vi "HIDRA.vi"() -> ()   [LabVIEW 2017]
uses:
  Type_Defs/Control.ctl
  Type_Defs/Diagnostics.ctl
  Type_Defs/Systems.ctl
  Type_Defs/Data.ctl
  Type_Defs/States.ctl
panel:
  out "Data Collecting?":bool
  in  "Data":T1
  out "Pressure":dbl format="%#.3g"
  out "Systems":T3
  out "Experiment State":T4(ring)
  out "Experiment Purpose":string
  out "Diagnostics":T2
  out "Step Number":i32
  out "Current Step Instructions":string
  in  "Controls":T5
  out "Time Elapsed":string
  out "Current Time":timestamp format="%<%X\n%x>T"
  out "Start Time":timestamp format="%<%X\n%x>T"
  out "Experiment Number":i32
  out "Operator":string
  # "HIDRA Control System"
  # "User Controls"
  # "Diagnostics"
  # "IGNORE PRESSURE AND SYSTEMS READINGS; NOT SET UP YET"
  # "Experiment Information"
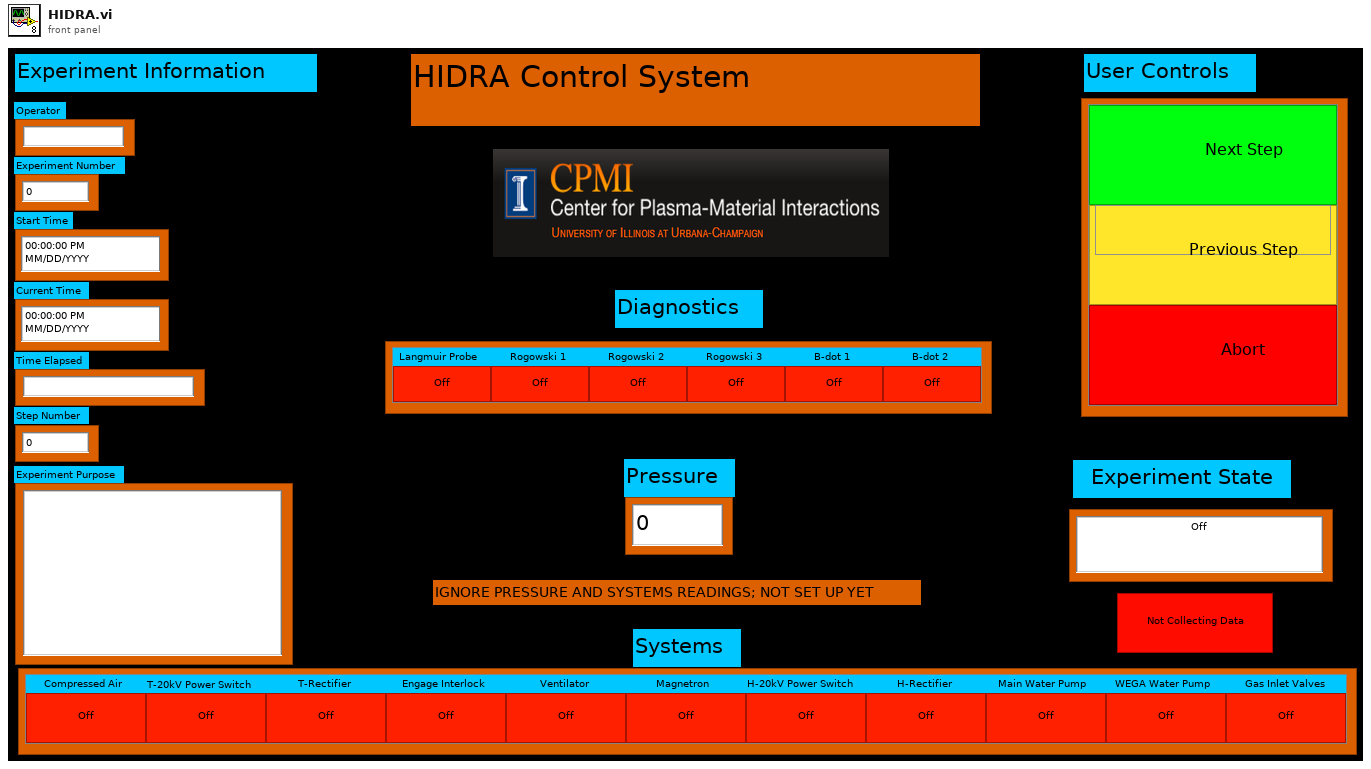
[diagram p1: front panel]
types:
  T1 = typedef "Data.ctl" = cluster{"User Name":string, "Experiment Number":i32, "Start Time":timestamp, "Data":dbl[], "Step Number":i32, "Step Instructions":string, "Diagnostics":T2, "Experiment Purpose":string, "Experiment State":enum16{"Off", "Setting Up", "Ready", "In Progress", "Shutting Down"}, "Systems":T3, "Vacuum Pressure":dbl, "Fieldpoints":cluster{"System Boolean Fieldpoints":cluster{"Compressed Air":refnum<k21>, "T-20kV Power Switch":refnum<k21>, "T-Rectifier":refnum<k21>, "Engage Interlock":refnum<k21>, "Ventilator":refnum<k21>, "Magnetron":refnum<k21>, "H-20kV Power Switch":refnum<k21>, "H-Rectifier":refnum<k21>, "Main Water Pump":refnum<k21>, "WEGA Water Pump":refnum<k21>, "Gas Inlet Valves":refnum<k21>}, "Step Fieldpoints":cluster{"Exhaust Ventillator":refnum<k21>, "Compressed Air":refnum<k21>, "Water Pressure":refnum<k21>, "Interlock":refnum<k21>, "Toroidal Power Supply 1":refnum<k21>, "Toroidal Power Supply 2":refnum<k21>, "Toroidal Rectifier":refnum<k21>, "Helical Power Supply":refnum<k21>, "Helical Rectifier":refnum<k21>, "6kW Magnetron Standby":refnum<k21>, "20kW Magnetron Standby":refnum<k21>}}, "Pressure History":cluster{"Seconds into Experiment":i32[], "Pressure Data":dbl[]}, "Time Computer Control":dbl[], "Toroidal Voltage Computer Control":dbl[], "Helical Voltage Computer Control":dbl[], "Toroidal Current":dbl[], "Toroidal Voltage":dbl[], "Toroidal Current Set Point":dbl[], "Helical Current Set Point":dbl[], "Helical Voltage":dbl[], "Helical Current":dbl[], "Experiment Folder":path, "Run Another Shot?":bool}
  T2 = typedef "Diagnostics.ctl" = cluster{"Langmuir Probe":bool, "Rogowski 1":bool, "Rogowski 2":bool, "Rogowski 3":bool, "B-dot 1":bool, "B-dot 2":bool}
  T3 = typedef "Systems.ctl" = cluster{"Compressed Air":bool, "T-20kV Power Switch":bool, "T-Rectifier":bool, "Engage Interlock":bool, "Ventilator":bool, "Magnetron":bool, "H-20kV Power Switch":bool, "H-Rectifier":bool, "Main Water Pump":bool, "WEGA Water Pump":bool, "Gas Inlet Valves":bool}
  T4 = enum16{"Off", "Setting Up", "Ready", "In Progress", "Shutting Down"}
  T5 = typedef "Control.ctl" = cluster{"Next Step":bool, "Previous Step":bool, "Abort":bool}
  T6 = typedef "States.ctl" = enum16{"1. Initialize", "2. User Information", "3. Experiment Information", "4. Create Data File", "5. Steps for Setup", "6. Gather Data", "7. Write to Data File", "8. Final", "Stop Pressed - Shutdown State"}
  T7 = enum8{"Enabled", "Disabled", "Disabled and Grayed Out"}
  T8 = enum32{"Invalid", "Standard", "Closed", "Hidden", "Minimized", "Maximized"}
  T9 = enum16{"open", "replace", "create", "open or create", "replace or create", "replace or create with confirmation"}
  T10 = enum16{"Always On", "Always Off", "Off While Running"}
  T11 = cluster{"Seconds into Experiment":i32[], "Pressure Data":dbl[]}
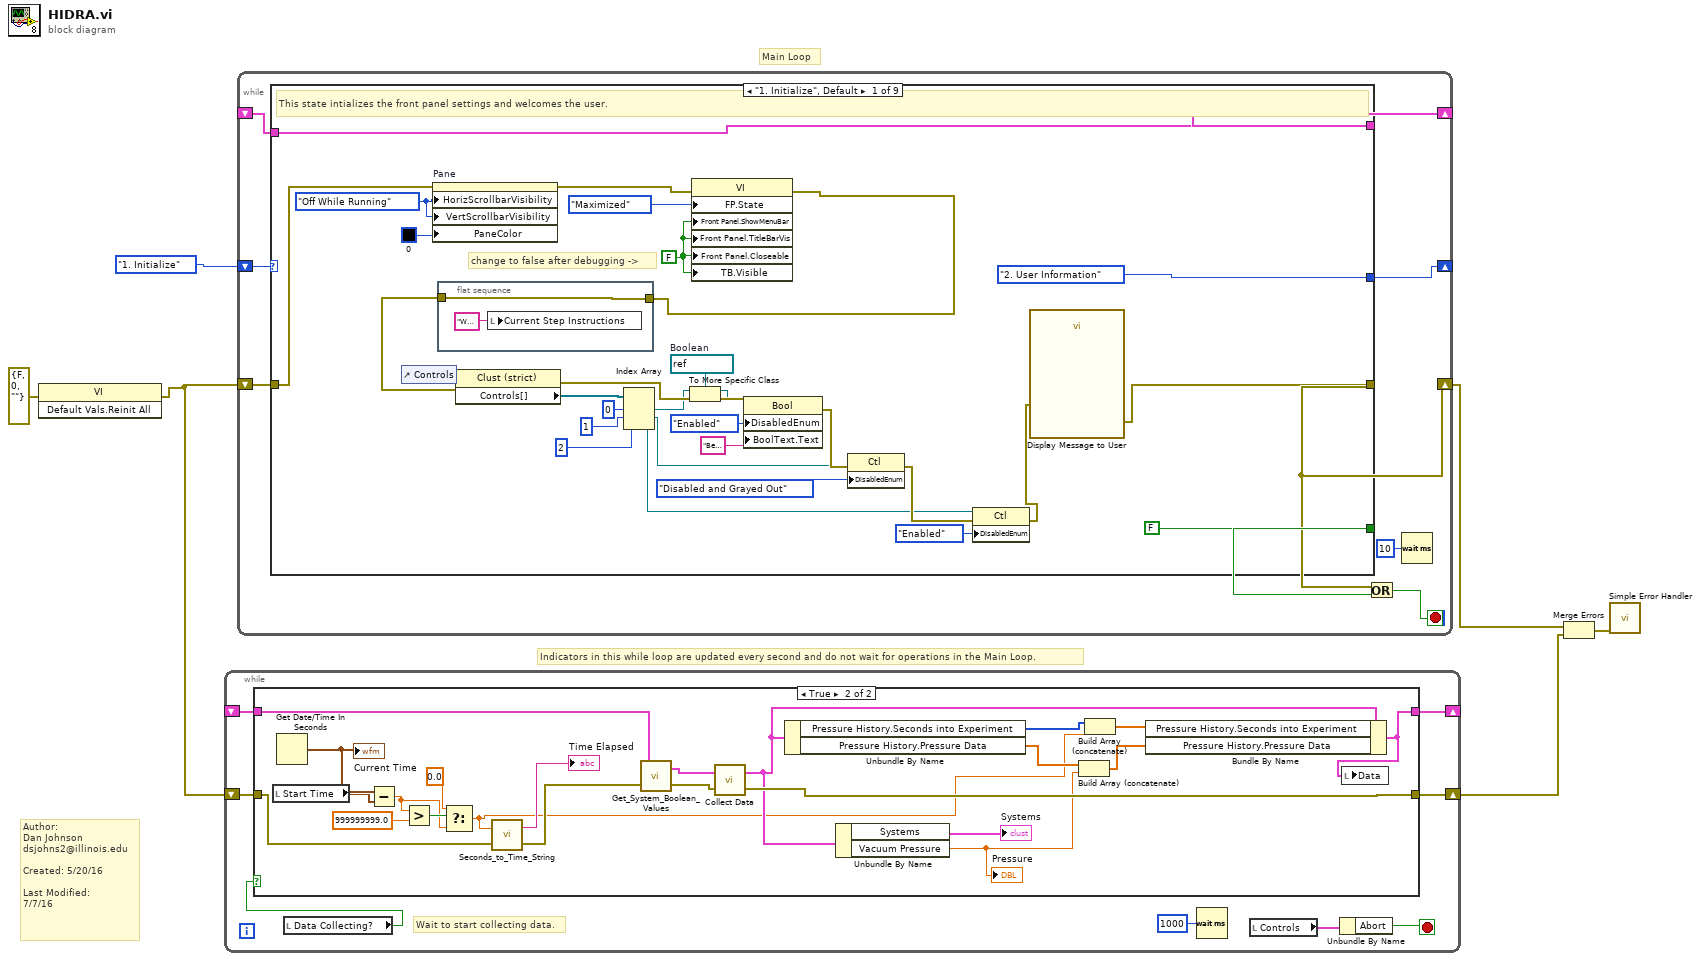
[diagram p0: block diagram]
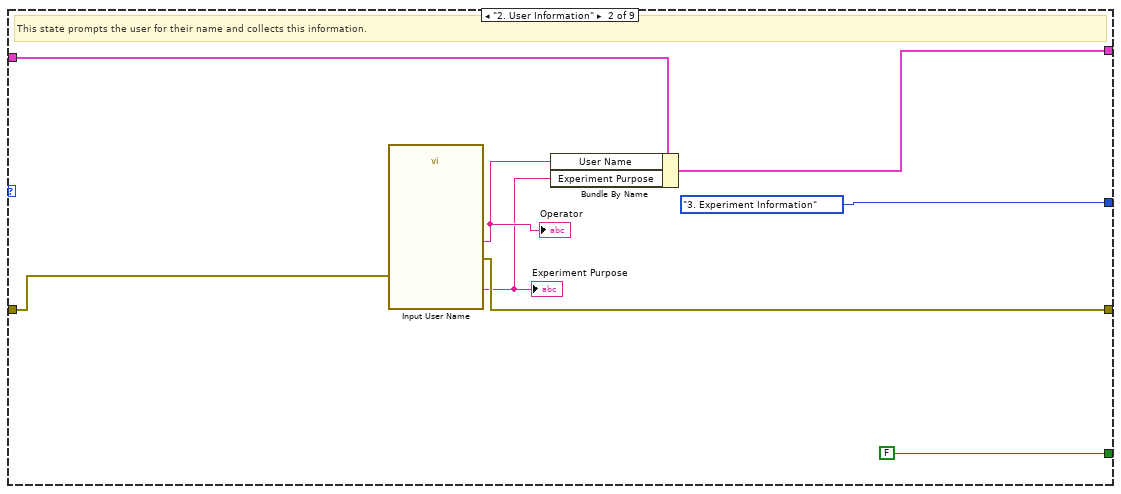
[diagram p3: hidden frame]
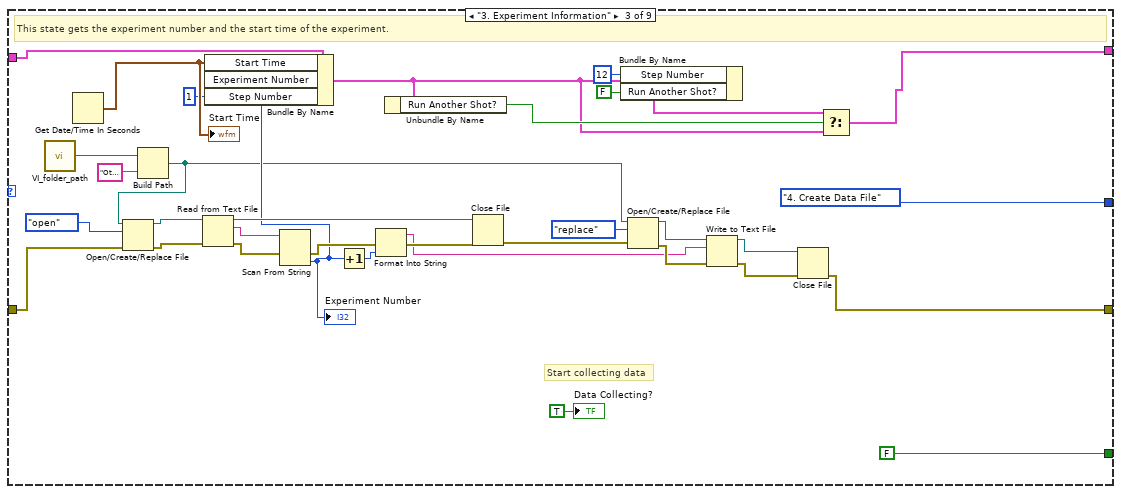
[diagram p4: hidden frame]
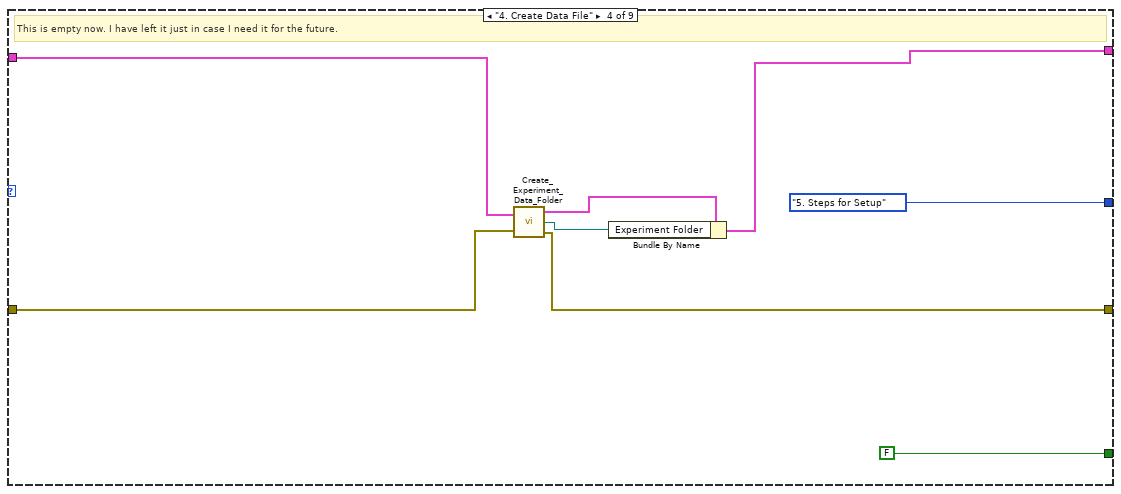
[diagram p5: hidden frame]
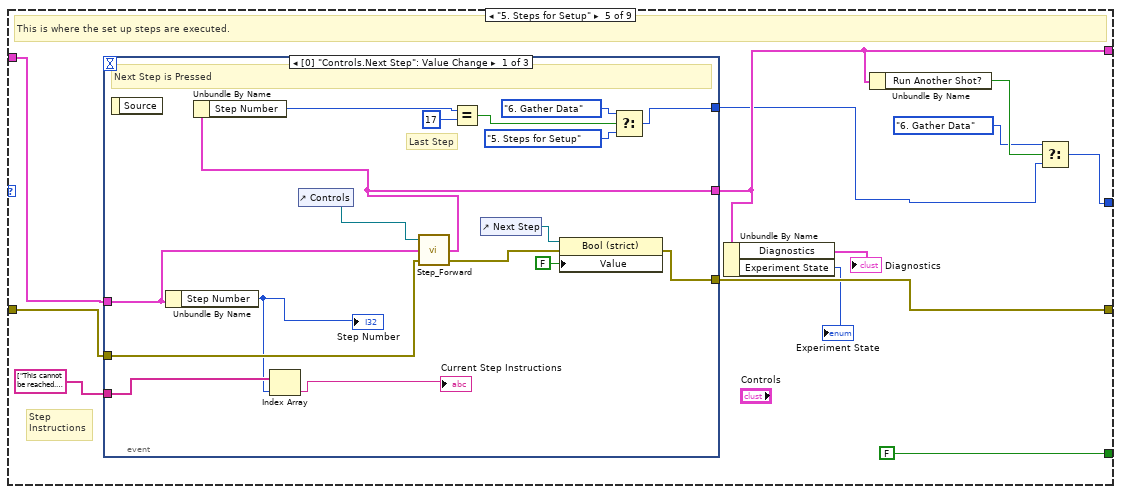
[diagram p6: hidden frame]
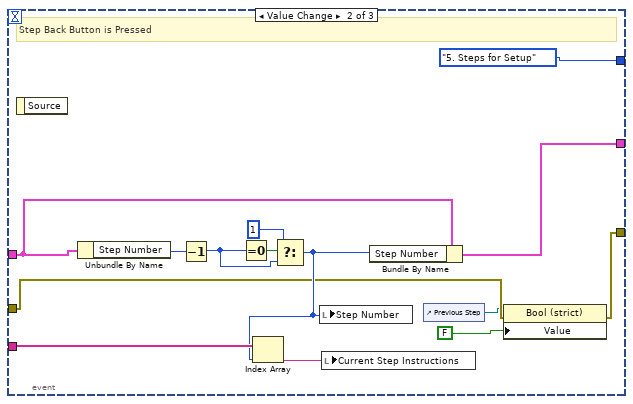
[diagram p7: hidden frame]
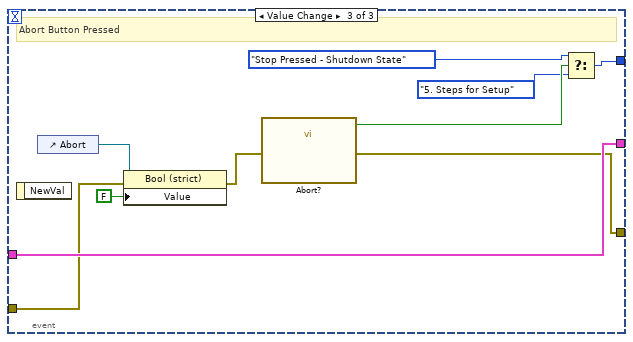
[diagram p8: hidden frame]
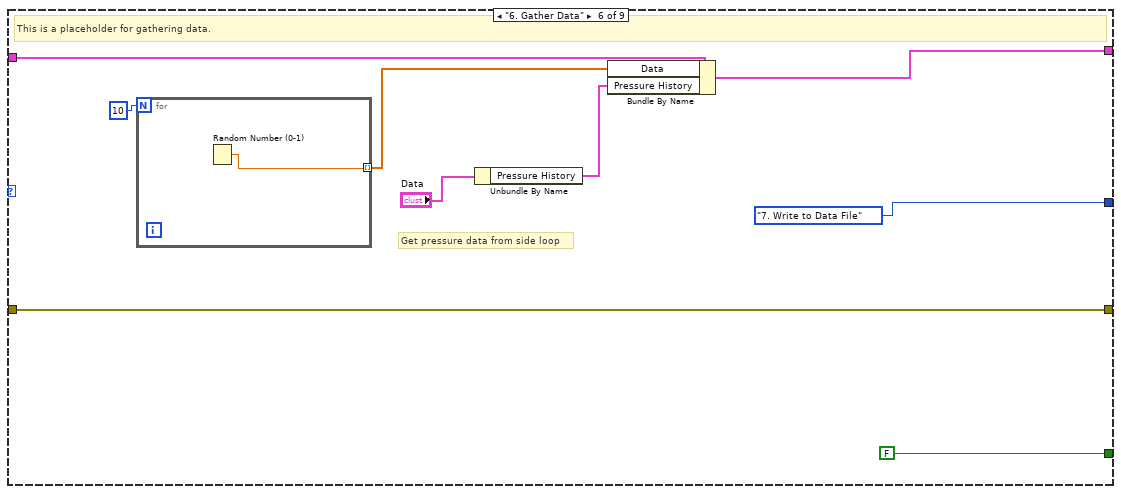
[diagram p9: hidden frame]
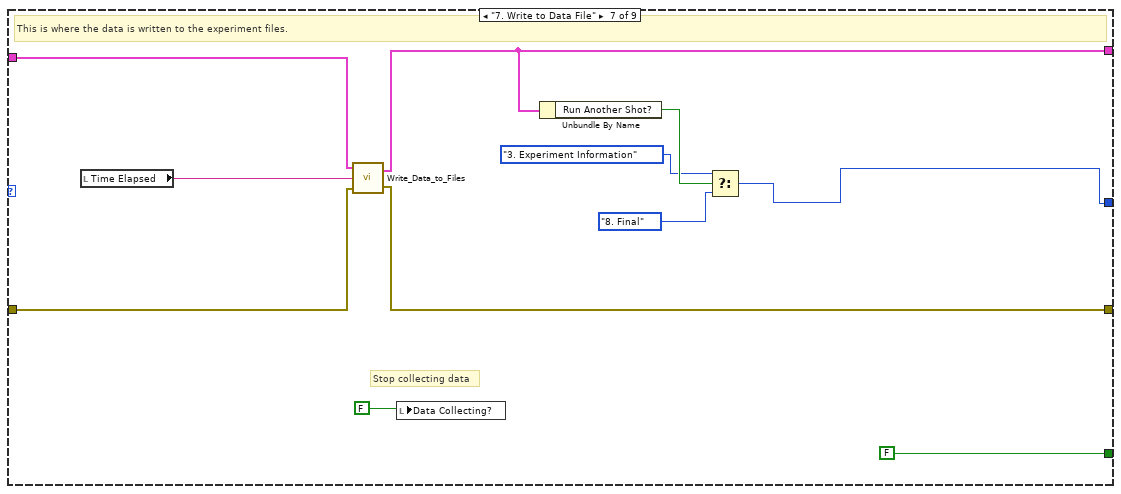
[diagram p10: hidden frame]
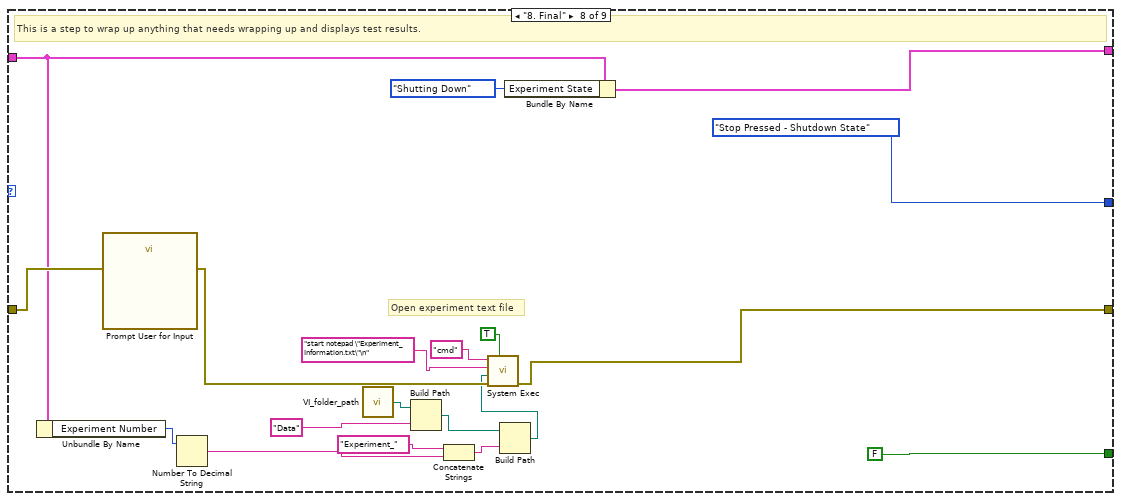
[diagram p11: hidden frame]
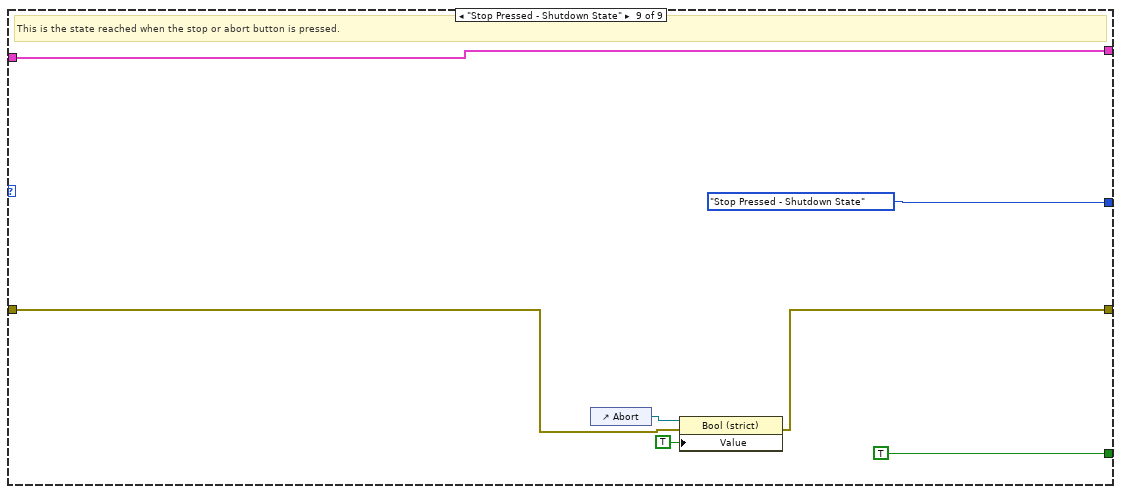
[diagram p12: hidden frame]
diagram:
  # "Main Loop"
  # "Indicators in this while loop are updated every second and do not wait for operations in the Main Loop."
  # "Author:\nDan Johnson\ndsjohns2@illinois.edu\n\nCreated: 5/20/16\n\nLast Modified:\n7/7/16"
  n1 = invoke class="VI" method="Default Vals.Reinit All"(error in=errorcluster {"status"=FALSE, "code"=0, "source"=""} ("error in (no error)")) -> (error out=w2:errorcluster)  [unwired: 2 in, 2 out]
  n2 = while {
    shift-right: [w13] -> w4
    shift-left: w2 -> [w12]
    shift-right: [w8] -> _
    shift-left: _ -> [w9]
    stop <- w10 stop-if-true
    # "Wait to start collecting data."
    n3 = local read "Data Collecting?"() -> (w7:bool)
    n4 = case shown="True" w7 {
      tunnel: [w16 w35] -> w13
      tunnel: w12 -> [w16 w18]
      tunnel: w9 -> [w15 w26]
      tunnel: [w15 w24] -> w8
      frame False {
      }
      frame True {
        n5 = local read "Start Time"() -> (w32:timestamp)
        n6 = Get Date/Time In Seconds() -> (seconds since 1Jan1904=w33:timestamp)
        "Current Time" <- w33
        n7 = Subtract(x=w33, y=w32) -> (x-y=w28:dbl)
        n8 = Greater?(x=w28, y=999999999.0) -> (0:w29:bool)
        n9 = Select(t=0.0, s=w29, f=w28) -> (s? t:f=w17:dbl)
        n10 = call "Seconds_to_Time_String.vi"("error in"=w18, "Seconds in"=w17) -> ("error out"=w34:errorcluster, "String"=→"Time Elapsed":string)
        n11 = call "Get_System_Boolean_Values.vi"("error in"=w34, "Data in"=w26) -> ("error out"=w37:errorcluster, "Data out"=w38:T1)
        n12 = call "Collect Data.vi"("error constant"=w37, "Data in"=w38) -> ("error constant 2"=w35:errorcluster, "Data out"=w25:T1)
        n13 = Unbundle By Name(w25) -> ("Pressure History.Seconds into Experiment"=w23:i32[], "Pressure History.Pressure Data"=w20:dbl[])
        n14 = Unbundle By Name(w25) -> ("Systems"=→"Systems":T3, "Vacuum Pressure"=w19:dbl)
        "Pressure" <- w19
        n15 = Build Array (concatenate)(w20, w19) -> (w21:dbl[])
        n16 = Build Array (concatenate)(w23, w17) -> (w22:dbl[])
        n17 = Bundle By Name(cluster=w25, "Pressure History.Seconds into Experiment"=w22, "Pressure History.Pressure Data"=w21) -> (w24:T1)
        n18 = local write "Data"(w24) -> ()
      }
    }
    n19 = Wait (ms)(milliseconds to wait=u32 1000) -> ()  [unwired: 1 out]
    n20 = local read "Controls"() -> (w11:T5)
    n21 = Unbundle By Name(w11) -> ("Abort"=w10:bool)
  }
  n22 = while {
    shift-right: [w39] -> _
    shift-left: States."1. Initialize" ("Enum") -> [w41]
    shift-right: [w40] -> _
    shift-left: _ -> [w46]
    shift-right: [w42] -> w5
    shift-left: w2 -> [w47]
    stop <- w44 stop-if-true
    n23 = case shown="\"1. Initialize\", Default" w41 {
      tunnel: w47 -> [w72 w86 w120 w127 w137 w186 w202 w219 w224]
      tunnel: w46 -> [w78 w84 w101 w128 w141 w191 w200 w214 w229]
      tunnel: [w78 w83 w93 w124 w135 w187 w196 w221 w229] -> w40
      tunnel: [FALSE FALSE FALSE FALSE FALSE FALSE FALSE FALSE TRUE] -> w43
      tunnel: [w71 w85 w100 w126 w140 w186 w201 w205 w225] -> w42
      tunnel: [States."2. User Information" ("Enum") States."3. Experiment Information" ("Enum") States."4. Create Data File" ("Enum") States."5. Steps for Setup" ("Enum") w131 States."7. Write to Data File" ("Enum") w194 States."Stop Pressed - Shutdown State" ("Enum") States."Stop Pressed - Shutdown State" ("Enum")] -> w39
      frame "1. Initialize", Default {
        w50 = refnum<vi> refnum  # Boolean
        w70 = FALSE
        w74 = T10."Off While Running" ("Vertical Scrollbar Visibility")
        # "change to false after debugging ->"
        # "This state intializes the front panel settings and welcomes the user."
        n24 = control-ref of="Controls"() -> (w68:refnum<vi>)
        n25 = property on="Pane" class="Pane"(error in=w72, "HorizScrollbarVisibility"=w74, "VertScrollbarVisibility"=w74, "PaneColor"=u32 0) -> (error out=w75:errorcluster)  [unwired: 1 in, 1 out]
        n26 = flat-sequence {
          tunnel: [w80] -> w55
          tunnel: w48 -> [w80]
          frame #0 {
            n27 = local write "Current Step Instructions"("Welcome to the Hybrid Illinois Device for Research and Applications (HIDRA)!" ("Current Step Instructions")) -> ()
          }
        }
        n28 = property class="Clust (strict)"(reference=w68, error in=w55) -> (error out=w54:errorcluster, "Controls[]"=w57:refnum<vi>[])  [unwired: 1 out]
        n29 = Index Array(array=w57, index #1=0 ("index"), index #2=1 ("index"), index #3=2 ("index")) -> (element #1=w52:refnum<vi>, element #2=w61:refnum<vi>, element #3=w62:refnum<vi>)
        n30 = To More Specific Class(target class=w50, reference=w52, error in=w54) -> (specific class reference=w51:refnum<vi>, error out=w53:errorcluster)
        n31 = property class="VI"(error in=w75, "FP.State"=T8."Maximized" ("Front Panel Window:State"), "Front Panel.ShowMenuBar"=w70, "Front Panel.TitleBarVis"=w70, "Front Panel.Closeable"=w70, "TB.Visible"=w70) -> (error out=w48:errorcluster)  [unwired: 1 in, 1 out]
        n32 = property class="Bool"(reference=w51, error in=w53, "DisabledEnum"=T7."Enabled" ("Disabled"), "BoolText.Text"="Begin Setup Steps" ("Boolean Text.Text")) -> (error out=w63:errorcluster)  [unwired: 1 out]
        n33 = property class="Ctl"(reference=w61, error in=w63, "DisabledEnum"=T7."Disabled and Grayed Out" ("Disabled")) -> (error out=w64:errorcluster)  [unwired: 1 out]
        n34 = property class="Ctl"(reference=w62, error in=w64, "DisabledEnum"=T7."Enabled" ("Disabled")) -> (error out=w56:errorcluster)  [unwired: 1 out]
        n35 = call "Display Message to User"("error in (no error)"=w56) -> ("error out"=w71:errorcluster)  [unwired: 9 in, 1 out]
      }
      frame "2. User Information" {
        # "This state prompts the user for their name and collects this information."
        n36 = call "Input User Name"("error in (no error)"=w86) -> ("Experiment Purpose"=w81:string, "User Name"=w88:string, "error out"=w85:errorcluster)  [unwired: 15 in, 1 out]
        "Operator" <- w88
        "Experiment Purpose" <- w81
        n37 = Bundle By Name(cluster=w84, "User Name"=w88, "Experiment Purpose"=w81) -> (w83:T1)
      }
      frame "3. Experiment Information" {
        # "Start collecting data"
        # "This state gets the experiment number and the start time of the experiment."
        n38 = call "VI_folder_path.vi"() -> ("output path"=w99:path)
        n39 = Get Date/Time In Seconds() -> (seconds since 1Jan1904=w103:timestamp)
        "Start Time" <- w103
        n40 = Build Path(base path=w99, name or relative path="Other\\Experiment_Number.txt") -> (appended path=w97:path)
        n41 = Open/Create/Replace File(file path (use dialog)=w97, error in=w120, operation (0:open)=T9."open") -> (refnum out=w112:refnum<file>, error out=w119:errorcluster)  [unwired: 3 in, 1 out]
        n42 = Read from Text File(file (use dialog)=w112, error in=w119) -> (refnum out=w111:refnum<file>, text=w107:string, error out=w118:errorcluster)  [unwired: 2 in, 1 out]
        n43 = Scan From String(input string=w107, error in=w118) -> (error out=w117:errorcluster, output 1=w104:i32)  [unwired: 3 in, 2 out]
        "Experiment Number" <- w104
        n44 = Bundle By Name(cluster=w101, "Start Time"=w103, "Experiment Number"=w104, "Step Number"=1) -> (w91:T1)
        n45 = Increment(x=w104) -> (x+1=w106:i32)
        n46 = Format Into String(error in=w117, w106) -> (resulting string=w105:string, error out=w116:errorcluster)  [unwired: 2 in]
        n47 = Unbundle By Name(w91) -> ("Run Another Shot?"=w94:bool)
        n48 = Close File(refnum=w111, error in=w116) -> (error out=w115:errorcluster)  [unwired: 1 out]
        n49 = Bundle By Name(cluster=w91, "Step Number"=12, "Run Another Shot?"=FALSE) -> (w92:T1)
        n50 = Open/Create/Replace File(file path (use dialog)=w97, error in=w115, operation (0:open)=T9."replace") -> (refnum out=w110:refnum<file>, error out=w114:errorcluster)  [unwired: 3 in, 1 out]
        n51 = Write to Text File(file (use dialog)=w110, text=w105, error in=w114) -> (refnum out=w109:refnum<file>, error out=w113:errorcluster)  [unwired: 1 in, 1 out]
        n52 = Close File(refnum=w109, error in=w113) -> (error out=w100:errorcluster)  [unwired: 1 out]
        n53 = Select(t=w92, s=w94, f=w91) -> (s? t:f=w93:T1)
        "Data Collecting?" <- TRUE ("Is Data")
      }
      frame "4. Create Data File" {
        # "This is empty now. I have left it just in case I need it for the future."
        n54 = call "Create_Experiment_Data_Folder.vi"("Data in"=w128, "error in"=w127) -> ("Data out"=w125:T1, "Folder path"=w123:path, "error out"=w126:errorcluster)
        n55 = Bundle By Name(cluster=w125, "Experiment Folder"=w123) -> (w124:T1)
      }
      frame "5. Steps for Setup" {
        # "Step\nInstructions"
        # "This is where the set up steps are executed."
        n56 = event shown="[0] \"Controls.Next Step\": Value Change" {
          selector: _ -> [_ _ _]
          dyn-events: _ -> [_ _ _]
          timeout: _ -> [_ _ _]
          tunnel: [w143 States."5. Steps for Setup" ("Enum") w181] -> w132
          tunnel: [w151 w163 w182] -> w140
          tunnel: w141 -> [w157 w172 w183]
          tunnel: [w155 w171 w183] -> w135
          tunnel: string[] ["This cannot be reached.", "This step sets up the step controls.", "Select the Diagnostics to be used.", "This step checks that the Vacuum Pressure is at the right value.", "This step checks that exhaust ventillator is operational.", "This step checks that the compressed air pressure is high enough.", "This step checks that the water pressure is high enough.", "This step checks that the interlock is on.", "This step checks that the toroidal power supply is on.", "This step checks that the toroidal rectifier is on.", "This step checks that the helical power supply is on.", "This step checks that the helical rectifier is on.", "This step sets the magnetron to standby mode.", "This step performs a final check to make sure everything is ready.", "This step does the following:\n  -Starts the Ramp Generator\n  -Opens the Gas Valve\n  -Resets the Radiation Detector", "This step sets up the pulse.", "This step is the pulse."] ("array") -> [w159 w169 _]
          tunnel: w137 -> [w156 w162 w177]
          event Value Change {
            # "Last Step"
            # "Next Step is Pressed"
            n57 = event-data() -> ()  [unwired: 1 in, 1 out]
            n58 = Unbundle By Name(w157) -> ("Step Number"=w154:i32)
            "Step Number" <- w154
            n59 = Index Array(array=w159, index=w154) -> (element=→"Current Step Instructions":string)
            n60 = control-ref of="Controls"() -> (w158:refnum<vi>)
            n61 = call "Step_Forward.vi"("error in"=w156, "Data in"=w157, "Step control reference in"=w158) -> ("error out"=w152:errorcluster, "Data out"=w155:T1)  [unwired: 1 out]
            n62 = Unbundle By Name(w155) -> ("Step Number"=w147:i32)
            n63 = Equal?(x=w147, y=17) -> (x = y?=w146:bool)
            n64 = control-ref of="Next Step"() -> (w150:refnum<vi>)
            n65 = property class="Bool (strict)"(reference=w150, error in=w152, "Value"=FALSE) -> (error out=w151:errorcluster)  [unwired: 1 out]
            n66 = Select(t=States."6. Gather Data" ("Enum"), s=w146, f=States."5. Steps for Setup" ("Enum")) -> (s? t:f=w143:T6)
          }
          event Value Change {
            # "Step Back Button is Pressed"
            n67 = event-data() -> ()  [unwired: 1 in, 1 out]
            n68 = Unbundle By Name(w172) -> ("Step Number"=w173:i32)
            n69 = Decrement(x=w173) -> (x-1=w165:i32)
            n70 = Equal To 0?(x=w165) -> (x = 0?=w167:bool)
            n71 = Select(t=1, s=w167, f=w165) -> (s? t:f=w164:i32)
            n72 = Index Array(array=w169, index=w164) -> (element=w170:string)
            n73 = local write "Step Number"(w164) -> ()
            n74 = local write "Current Step Instructions"(w170) -> ()
            n75 = Bundle By Name(cluster=w172, "Step Number"=w164) -> (w171:T1)
            n76 = control-ref of="Previous Step"() -> (w160:refnum<vi>)
            n77 = property class="Bool (strict)"(reference=w160, error in=w162, "Value"=FALSE) -> (error out=w163:errorcluster)  [unwired: 1 out]
          }
          event Value Change {
            # "Abort Button Pressed"
            n78 = event-data() -> ()  [unwired: 1 in, 1 out]
            n79 = control-ref of="Abort"() -> (w175:refnum<vi>)
            n80 = property class="Bool (strict)"(reference=w175, error in=w177, "Value"=FALSE) -> (error out=w176:errorcluster)  [unwired: 1 out]
            n81 = call "Abort?"("error in (no error)"=w176) -> ("Abort"=w180:bool, "error out"=w182:errorcluster)  [unwired: 17 in]
            n82 = Select(t=States."Stop Pressed - Shutdown State" ("Enum"), s=w180, f=States."5. Steps for Setup") -> (s? t:f=w181:T6)
          }
        }
        n83 = Unbundle By Name(w135) -> ("Diagnostics"=→"Diagnostics":T2, "Experiment State"=→"Experiment State":T4)
        n84 = Unbundle By Name(w135) -> ("Run Another Shot?"=w134:bool)
        n85 = Select(t=States."6. Gather Data" ("Enum"), s=w134, f=w132) -> (s? t:f=w131:T6)
      }
      frame "6. Gather Data" {
        # "Get pressure data from side loop"
        # "This is a placeholder for gathering data."
        n86 = for {
          N: 10 -> [_]
          tunnel: [w193] -> w190 mode=indexing
          n87 = Random Number (0-1)() -> (number: 0 to 1=w193:dbl)
        }
        n88 = Unbundle By Name("Data") -> ("Pressure History"=w185:T11)
        n89 = Bundle By Name(cluster=w191, "Data"=w190, "Pressure History"=w185) -> (w187:T1)
      }
      frame "7. Write to Data File" {
        # "Stop collecting data"
        # "This is where the data is written to the experiment files."
        n90 = local read "Time Elapsed"() -> (w203:string)
        n91 = call "Write_Data_to_Files.vi"("error in"=w202, "Time Elapsed"=w203, "Data in"=w200) -> ("error out"=w201:errorcluster, "Data out"=w196:T1)
        n92 = local write "Data Collecting?"(FALSE ("Is Data")) -> ()
        n93 = Unbundle By Name(w196) -> ("Run Another Shot?"=w198:bool)
        n94 = Select(t=States."3. Experiment Information" ("Enum"), s=w198, f=States."8. Final" ("Enum")) -> (s? t:f=w194:T6)
      }
      frame "8. Final" {
        # "Open experiment text file"
        # "This is a step to wrap up anything that needs wrapping up and displays test results."
        n95 = Unbundle By Name(w214) -> ("Experiment Number"=w213:i32)
        n96 = call "Prompt User for Input"("error in (no error)"=w219) -> ("error out"=w218:errorcluster)  [unwired: 17 in, 1 out]
        n97 = Number To Decimal String(number=w213) -> (decimal integer string=w206:string)  [unwired: 1 in]
        n98 = call "VI_folder_path.vi"() -> ("output path"=w215:path)
        n99 = Build Path(base path=w215, name or relative path="Data") -> (appended path=w212:path)
        n100 = Concatenate Strings("Experiment_" ("string"), w206) -> (w209:string)
        n101 = Build Path(base path=w212, name or relative path=w209) -> (appended path=w208:path)
        n102 = call <vilib>:"System Exec.vi"("wait until completion? (T)"=TRUE, "error in (no error)"=w218, "working directory"=w208, "standard input"="start notepad \"Experiment_Information.txt\"\n", "command line"="cmd") -> ("error out"=w205:errorcluster)  [unwired: 3 in, 3 out]
        n103 = Bundle By Name(cluster=w214, "Experiment State"=T4."Shutting Down") -> (w221:T1)
      }
      frame "Stop Pressed - Shutdown State" {
        # "This is the state reached when the stop or abort button is pressed."
        n104 = control-ref of="Abort"() -> (w227:refnum<vi>)
        n105 = property class="Bool (strict)"(reference=w227, error in=w224, "Value"=TRUE) -> (error out=w225:errorcluster)  [unwired: 1 out]
      }
    }
    n106 = Or(x=w42, y=w43) -> (x .or. y?=w44:bool)
    n107 = Wait (ms)(milliseconds to wait=u32 10) -> ()  [unwired: 1 out]
  }
  n108 = Merge Errors(w5, w4) -> (w3:errorcluster)
  n109 = call <vilib>:"Simple Error Handler.vi"("error in (no error)"=w3) -> ()  [unwired: 4 in, 5 out]
